vi "apply key value pairs.vi"(8 "error in":errorcluster, 9 "values":string[](array[string]), 10 "keys":string[](array[string]), 11 "fixed channel runtime in":refnum<class "MotionModule runtime.lvclass">) -> (0 "error out":errorcluster, 3 "fixed channel runtime out":refnum<class "MotionModule runtime.lvclass">)   [LabVIEW 2017, in "MotionModule runtime.lvclass"]
uses:
  MotionModule runtime.lvclass
  MotionModule runtime.lvclass/MotionModule runtime.ctl
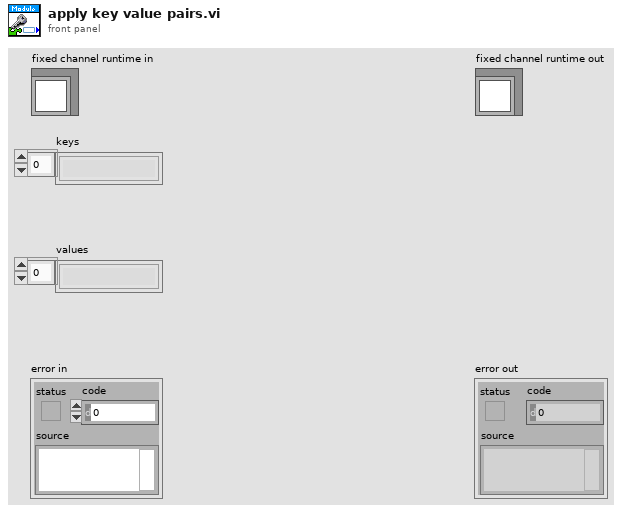
[diagram p1: front panel]
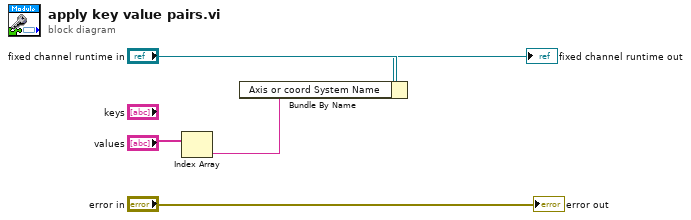
[diagram p0: block diagram]
diagram:
  n1 = Index Array(array="values") -> (element=w1:string)  [unwired: 1 in]
  n2 = Bundle By Name(cluster="fixed channel runtime in", "Axis or coord System Name"=w1) -> (→"fixed channel runtime out":refnum<class "MotionModule runtime.lvclass">)
  "error out" <- "error in"
